vi "Read Exception Status.vi"(7 "unit ID":u8, 8 "error in":errorcluster, 11 "Modbus slave in":refnum<class "Modbus Slave.lvclass">) -> (0 "error out":errorcluster, 2 "exception status":u8, 3 "Modbus slave out":refnum<class "Modbus Slave.lvclass">)   [LabVIEW 2013, in "Modbus Library - Advance.lvlib" / "Modbus Slave.lvclass"]
doc: "Interface to reads any exception status set in the device. The exeption status is a set of 8 status bits, packed as a U8 integer. With third-party devices, this function should only be used if the device is a serial device, as the Modbus specification defines this as a serial-only function. However, this library includes support for this function regardless of the transport mechanism."
uses:
  Modbus Slave.lvclass
  Modbus Slave.lvclass/Modbus Slave.ctl
  Standard Data Model/Standard Data Model.lvclass
  Super Data Model/Super Data Model.lvclass
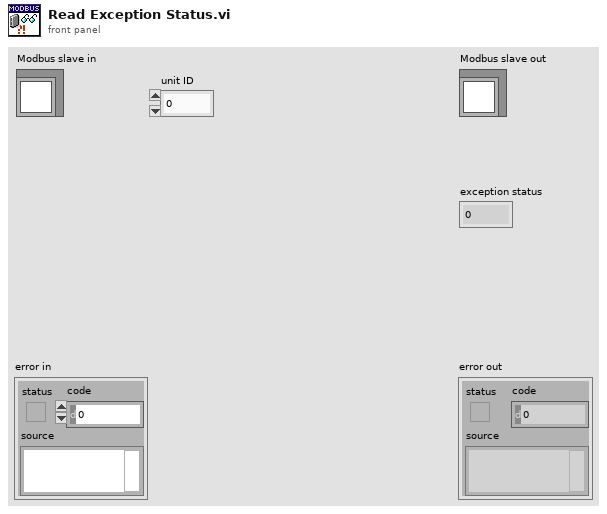
[diagram p1: front panel]
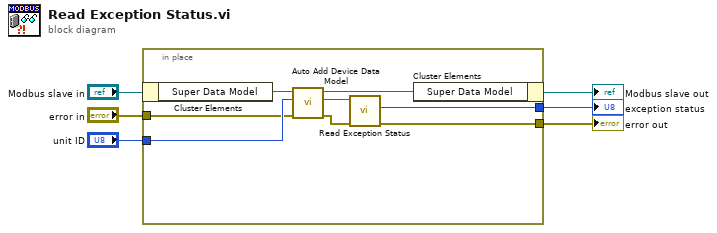
[diagram p0: block diagram]
diagram:
  n1 = in-place {
    in-place-border: [w14] -> w3
    in-place-border: [w13] -> w4
    in-place-border: "error in" -> [w10]
    in-place-border: "unit ID" -> [w11]
    n2 = in-place-cluster #1("Modbus slave in") -> ("Super Data Model"=w12:refnum<class "Super Data Model.lvclass">)
    n3 = call "Auto Add Device Data Model.vi"("error in"=w10, "unit ID"=w11, "Super Data Model in"=w12) -> ("error out"=w7:errorcluster, "device data model"=w8:refnum<class "Standard Data Model.lvclass">, "Super Data Model out"=w9:refnum<class "Super Data Model.lvclass">)  [unwired: 6 in]
    n4 = call-dynamic "Read Exception Status.vi"("error in"=w7, "device data model in"=w8) -> ("error out"=w13:errorcluster, "exception status"=w14:u8)  [unwired: 7 in, 1 out]
    n5 = in-place-cluster #1("Super Data Model"=w9) -> (→"Modbus slave out":refnum<class "Modbus Slave.lvclass">)
  }
  "error out" <- w4
  "exception status" <- w3
